vi "AuMT8852 Initialize with Options.vi"(7 "Options":T1, 8 "error in (no error)":errorcluster, 9 "Reset (T)":bool, 10 "ID Query (T)":bool, 11 "Resource descriptor (\"GPIB0::27\")":string="GPIB0::27") -> (0 "error out":errorcluster, 3 "VISA session out":refnum<visa-resource-name>)   [LabVIEW 2017]
doc: "Anritsu MT8852 Bluetooth Tester\n\nOpens a connection to the instrument.\n\nINPUTS\n Resource descriptor - describes how your PC will communicate to the instrument:\n For GPIB connection, use\n GPIB0::<address>\n For multiple GPIB cards, use\n GPIB<card>::<address>\n For serial connection, use\n ASRL<COM port number>::INSTR\n ID Query - whether or not the driver will check to make sure the instrument is an MT8850.\n Reset - whether or not the driver will reset the instrument to a known state.\n Options - set the behavior of the driver."
panel:
  # "For GPIB connection, use\nGPIB0::<address>\n\nFor multiple GPIB cards, use\nGPIB<card>::<address>\n\nFor serial connection, use\nASRL<COM port number>::INSTR"
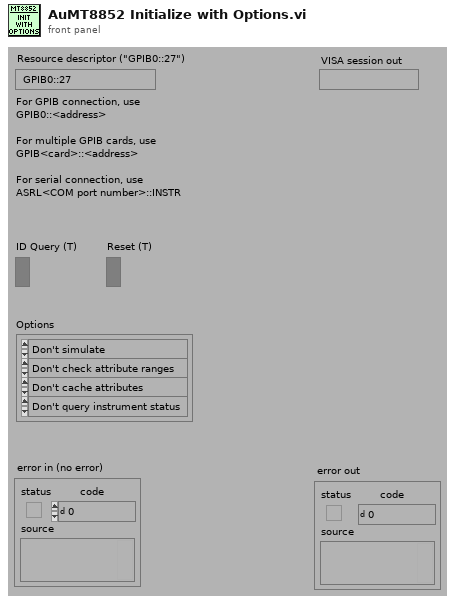
[diagram p1: front panel]
types:
  T1 = cluster{"Simulation":enum16{"Don't simulate", "Simulate"}, "Range checking":enum16{"Don't check attribute ranges", "Check attribute ranges"}, "State caching":enum16{"Don't cache attributes", "Cache attributes"}, "Status checking":enum16{"Don't query instrument status", "Query instrument status"}}
  T2 = cluster{"Simulate?":bool, "Range check?":bool, "Cache?":bool, "Query instrument status?":bool}
  T3 = enum16{"Don't check attribute ranges", "Check attribute ranges"}
  T4 = enum16{"Don't cache attributes", "Cache attributes"}
  T5 = enum16{"Don't query instrument status", "Query instrument status"}
  T6 = typedef "Instrument Object Reference.ctl" = refnum<k1>
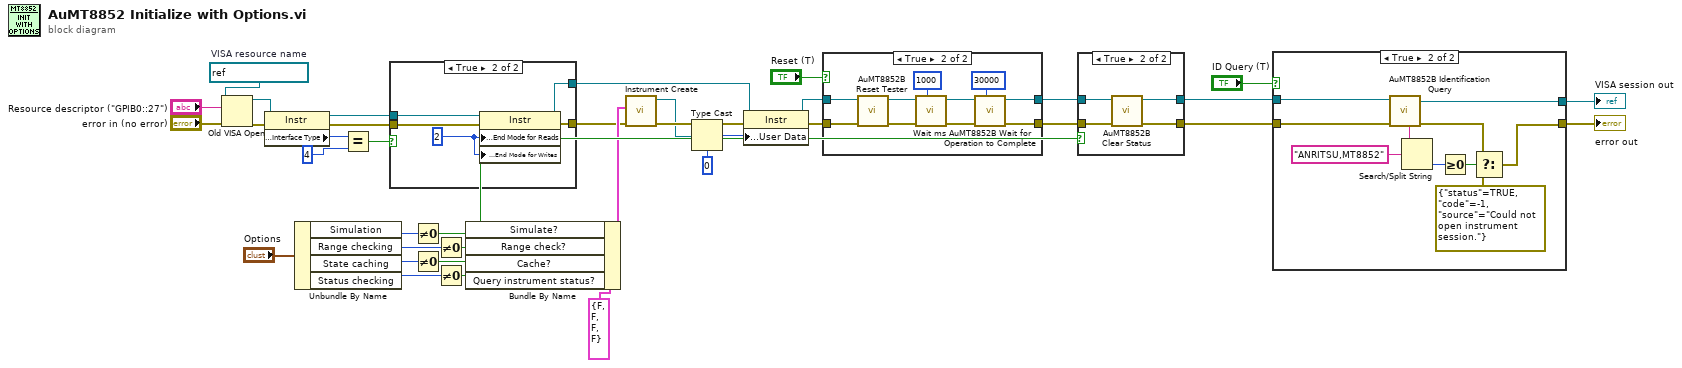
[diagram p0: block diagram]
diagram:
  w32 = refnum<visa-resource-name> refnum  # VISA resource name
  n1 = Old VISA Open(8:"error in (no error)", 10:"Resource descriptor (\"GPIB0::27\")", 11:w32) -> (0:w13:errorcluster, 3:w12:refnum<visa-resource-name>)  [unwired: 2 in]
  n2 = property class="Instr"(reference=w12, error in=w13) -> (reference out=w8:refnum<visa-resource-name>, error out=w7:errorcluster, "Interface Information:Interface Type"=w11:u16)
  n3 = Unbundle By Name("Options") -> ("Simulation"=w20:enum16{"Don't simulate", "Simulate"}, "Range checking"=w19:T3, "State caching"=w18:T4, "Status checking"=w17:T5)
  n4 = Equal?(x=w11, y=u16 4 ("Interface Information:Interface Type")) -> (x = y?=w9:bool)
  n5 = case shown="True" w9 {
    tunnel: w8 -> [w38 w44]
    tunnel: w7 -> [w39 w43]
    tunnel: [w39 w41] -> w6
    tunnel: [w38 w40] -> w5
    frame False {
    }
    frame True {
      w42 = u16 2 ("Serial Settings:Serial End Mode for Reads")
      n6 = property class="Instr"(reference=w44, error in=w43, "Serial Settings:End Mode for Reads"=w42, "Serial Settings:End Mode for Writes"=w42) -> (reference out=w40:refnum<visa-resource-name>, error out=w41:errorcluster)
    }
  }
  n7 = Not Equal To 0?(x=w20) -> (x != 0?=w30:bool)
  n8 = Not Equal To 0?(x=w18) -> (x != 0?=w28:bool)
  n9 = Not Equal To 0?(x=w19) -> (x != 0?=w29:bool)
  n10 = Not Equal To 0?(x=w17) -> (x != 0?=w27:bool)
  n11 = Bundle By Name(cluster=T2 {"Simulate?"=FALSE, "Range check?"=FALSE, "Cache?"=FALSE, "Query instrument status?"=FALSE} ("Input Cluster"), "Simulate?"=w30, "Range check?"=w29, "Cache?"=w28, "Query instrument status?"=w27) -> (w26:T2)
  n12 = call <instrlib>:"Instrument Create.vi"("error in (no error)"=w6, "IVI flags"=w26) -> ("error out"=w37:errorcluster, "reference"=w35:T6)  [unwired: 8 in]
  n13 = Type Cast(type=u32 0, x=w35) -> (*(type *) &x=w34:u32)
  n14 = property class="Instr"(reference=w5, error in=w37, "General Settings:User Data"=w34) -> (reference out=w24:refnum<visa-resource-name>, error out=w25:errorcluster)
  n15 = case shown="True" "Reset (T)" {
    tunnel: w25 -> [w45 w56]
    tunnel: w24 -> [w46 w55]
    tunnel: [w46 w50] -> w4
    tunnel: [w45 w49] -> w3
    frame False {
    }
    frame True {
      n16 = call <instrlib>:"AuMT8852B Reset Tester.vi"("error in (no error)"=w56, "VISA session"=w55) -> ("error out"=w54:errorcluster, "VISA session out"=w53:refnum<visa-resource-name>)  [unwired: 7 in, 1 out]
      n17 = call <instrlib>:"Wait ms.vi"("Wait (1000 ms)"=u32 1000, "error in (no error)"=w54, "VISA Session"=w53) -> ("error out"=w47:errorcluster, "VISA Session out"=w48:refnum<visa-resource-name>)  [unwired: 7 in]
      n18 = call <instrlib>:"AuMT8852B Wait for Operation to Complete.vi"("Timeout (10000 ms)"=30000, "error in (no error)"=w47, "VISA session"=w48) -> ("error out"=w49:errorcluster, "VISA session out"=w50:refnum<visa-resource-name>)  [unwired: 6 in, 1 out]
    }
  }
  n19 = case shown="True" w27 {
    tunnel: w3 -> [w57 w62]
    tunnel: w4 -> [w58 w61]
    tunnel: [w57 w60] -> w2
    tunnel: [w58 w59] -> w1
    frame False {
    }
    frame True {
      n20 = call <instrlib>:"AuMT8852B Clear Status.vi"("error in (no error)"=w62, "VISA session"=w61) -> ("error out"=w60:errorcluster, "VISA session out"=w59:refnum<visa-resource-name>)  [unwired: 7 in, 1 out]
    }
  }
  n21 = case shown="True" "ID Query (T)" {
    tunnel: w2 -> [w64 w74]
    tunnel: [w63 w73] -> w23
    tunnel: [w64 w68] -> w22
    tunnel: w1 -> [w63 w65]
    frame False {
    }
    frame True {
      n22 = call <instrlib>:"AuMT8852B Identification Query.vi"("error in (no error)"=w74, "VISA session"=w65) -> ("error out"=w66:errorcluster, "VISA session out"=w73:refnum<visa-resource-name>, "Identification"=w67:string)  [unwired: 6 in, 1 out]
      n23 = Search/Split String(string=w67, search string/char (-)="ANRITSU,MT8852") -> (offset of match=w71:i32)  [unwired: 1 in, 2 out]
      n24 = Greater Or Equal To 0?(x=w71) -> (x >= 0?=w70:bool)
      n25 = Select(t=w66, s=w70, f=errorcluster {"status"=TRUE, "code"=-1, "source"="Could not open instrument session."}) -> (s? t:f=w68:errorcluster)
    }
  }
  "error out" <- w22
  "VISA session out" <- w23
